vi "Periodic Tasks.vi"(8 "error in":errorcluster) -> ()   [LabVIEW 2016]
doc: "This VI runs in parallel to other tasks. It can contain as many user-defined periodic loops as you need. These can carry out PID or other sorts of timed response."
uses:
  <vilib>/Rock Robotics/WPI/Utilities/WPI_GetSetVariantRefNum.vi
  <vilib>/Rock Robotics/Network Tables/NT Write Number.vi
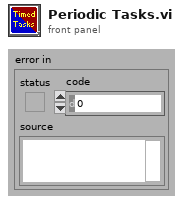
[diagram p1: front panel]
types:
  T1 = typedef "WPI_JoystickDevRef.ctl" = cluster{"Device":T2}
  T2 = typedef "WPI_JoystickDeviceEnum.ctl" = enum16{"USB 0", "USB 1", "USB 2", "USB 3", "USB 4", "USB 5"}
  T3 = typedef "WPI_RobotDriveDevRef.ctl" = cluster{"DevStatus":errorcluster, "Motors[]":T4[], "Square Inputs":bool, "Max Output":dbl}
  T4 = typedef "WPI_MotorControlDeviceRef.ctl" = cluster{"DeviceStatus":errorcluster, "Type":T5, "PWM":cluster{"PWM Channel":T6, "DeadBand":T7}, "CAN":cluster{"Device Number":u8, "SetOutput VI Ref":variant, "GetOutput VI Ref":variant, "Enable VI Ref":variant, "Disable VI Ref":variant, "Data":variant}, "Invert":bool}
  T5 = typedef "WPI_MotorControlType.ctl" = enum16{"PWM", "CAN"}
  T6 = typedef "FPGA_DIOPWMChannel.ctl" = enum8{"PWM 0", "PWM 1", "PWM 2", "PWM 3", "PWM 4", "PWM 5", "PWM 6", "PWM 7", "PWM 8", "PWM 9", "PWM MXP 0", "PWM MXP 1", "PWM MXP 2", "PWM MXP 3", "PWM MXP 4", "PWM MXP 5", "PWM MXP 6", "PWM MXP 7", "PWM MXP 8", "PWM MXP 9", "Invalid"}
  T7 = typedef "WPI_PWMDeadband.ctl" = cluster{"Name":string, "maxPositivePwm":i32, "minPositivePwm":i32, "centerPwm":i32, "maxNegativePwm":i32, "minNegativePwm":i32, "angularRange":u16}
  T8 = typedef "WPI_GyroDevRef.ctl" = cluster{"DevStatus":errorcluster, "Analog Channel":T9, "Offset":dbl, "Gain (VoltsPerDegree/Second)":dbl, "Gyro Type":enum16{"Analog", "XRS450"}, "Handle":i32, "SPI Bus":T10, "Device Found":bool, "Sample Rate":dbl, "Calibrate On Open":bool}
  T9 = typedef "FPGA_AIChannel.ctl" = enum8{"AI 0", "AI 1", "AI 2", "AI 3", "AI MXP 0", "AI MXP 1", "AI MXP 2", "AI MXP 3", "Invalid"}
  T10 = typedef "spi_bus.ctl" = enum16{"SPI On-Board, CS0", "SPI On-Board, CS1", "SPI On-Board, CS2", "SPI On-Board, CS3", "SPI MXP", "Invalid"}
  T11 = cluster{"JoystickDevRef":T1, "RobotDriveDevRef":T3, "GyroDevRef":T8}
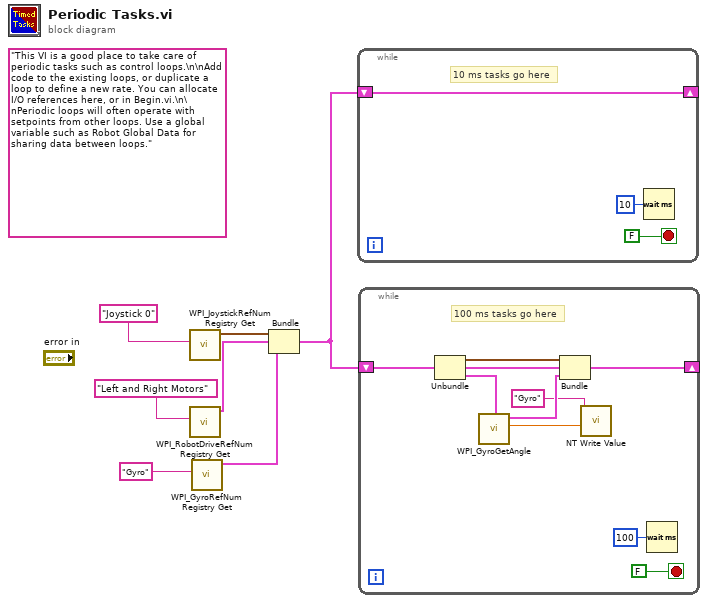
[diagram p0: block diagram]
diagram:
  (unwired) "This VI is a good place to take care of periodic tasks such as control loops.\n\nAdd code to the existing loops, or duplicate a loop to define a new rate. You can allocate I/O references here, or in Begin.vi.\n\nPeriodic loops will often operate with setpoints from other loops. Use a global variable such as Robot Global Data for sharing data between loops."
  n1 = call <vilib>:"WPI_JoystickRefNum Registry Get.vi"("refnum name"="Joystick 0") -> ("JoystickDevRef"=w5:T1)  [unwired: 1 in, 9 out]
  n2 = call <vilib>:"WPI_RobotDriveRefNum Registry Get.vi"("refnum name"="Left and Right Motors") -> ("RobotDriveDevRef"=w2:T3)  [unwired: 1 in, 9 out]
  n3 = call <vilib>:"WPI_GyroRefNum Registry Get.vi"("refnum name"="Gyro") -> ("GyroDevRef"=w1:T8)  [unwired: 9 in, 1 out]
  n4 = Bundle("JoystickDevRef"=w5, "RobotDriveDevRef"=w2, "GyroDevRef"=w1) -> (w4:T11)  [unwired: 1 out]
  n5 = while {
    shift-right: [w8] -> _
    shift-left: w4 -> [w8]
    stop <- FALSE stop-if-true
    # "10 ms tasks go here"
    n6 = Wait (ms)(milliseconds to wait=u32 10) -> ()  [unwired: 1 out]
  }
  n7 = while {
    shift-right: [w14] -> _
    shift-left: w4 -> [w19]
    stop <- FALSE stop-if-true
    # "100 ms tasks go here"
    n8 = Unbundle(w19) -> ("JoystickDevRef"=w16:T1, "RobotDriveDevRef"=w15:T3, "GyroDevRef"=w17:T8)
    n9 = call <vilib>:"WPI_GyroGetAngle.vi"("GyroDevRef"=w17) -> ("Angle"=w13:dbl, "GyroDevRef"=w12:T8)  [unwired: 6 in, 3 out]
    n10 = Bundle("JoystickDevRef"=w16, "RobotDriveDevRef"=w15, "GyroDevRef"=w12) -> (w14:T11)  [unwired: 1 in]
    n11 = call-poly <vilib>:"NT Write Value.vi"("Numeric"=w13, "Name"="Gyro") -> ()  [unwired: 9 in, 1 out]
    n12 = Wait (ms)(milliseconds to wait=u32 100) -> ()  [unwired: 1 out]
  }
